vi "Run.vi"(8 "error in (no error)":errorcluster, 11 "Switching Times in":refnum<class "Switching Time.lvclass">) -> (0 "error out":errorcluster, 1 "Parameters":cluster{"Name":string, "Value":string}[](array[cluster]), 2 "Canceled":bool, 3 "Switching Times out":refnum<class "Switching Time.lvclass">)   [LabVIEW 2020, in "Switching Time.lvclass"]
doc: "This is the main test vi. It is here that the test is implemented."
uses:
  Switching Time.lvclass
  C:/Sandbox/Git_Sandbox/WiSpry Test Framework source code (LV20)/WiSpry Test Framework/Measurements/Measurement.lvclass
  Controls/Run States.ctl
  Devices/Controls/Change setting mode enum.ctl
  Measurement.lvclass/Measurement.ctl
  XML Handler/Controls/Result Cluster.ctl
  XML Handler/XML Handler.lvclass/XML Handler.ctl
  Support VI/Update parameters (array).vi
  Support VI/Update parameters (single).vi
  <vilib>/Waveform/WDTFileIO.llb/Export Waveforms To Spreadsheet File (1D).vi
  Measurement.lvclass
  Instruments/Signal Generator/Signal Generator.lvclass
  Devices/Device.lvclass
  Instruments/Oscilloscope/Oscilloscope.lvclass
  Instruments/Spectrum Analyzer/Spectrum Analyzer.lvclass
  Devices/PIC-device/PIC-Device.lvclass
  Instruments/Power Supply/Power Supply.lvclass
  Instruments/Digital Multimeter/Digital Multimeter.lvclass
  XML Handler/XML Handler.lvclass
panel:
  out "resulting string":string
  out "Waveform Graph":waveform(dbl)[](graph)
  in  "Cancel Button":bool
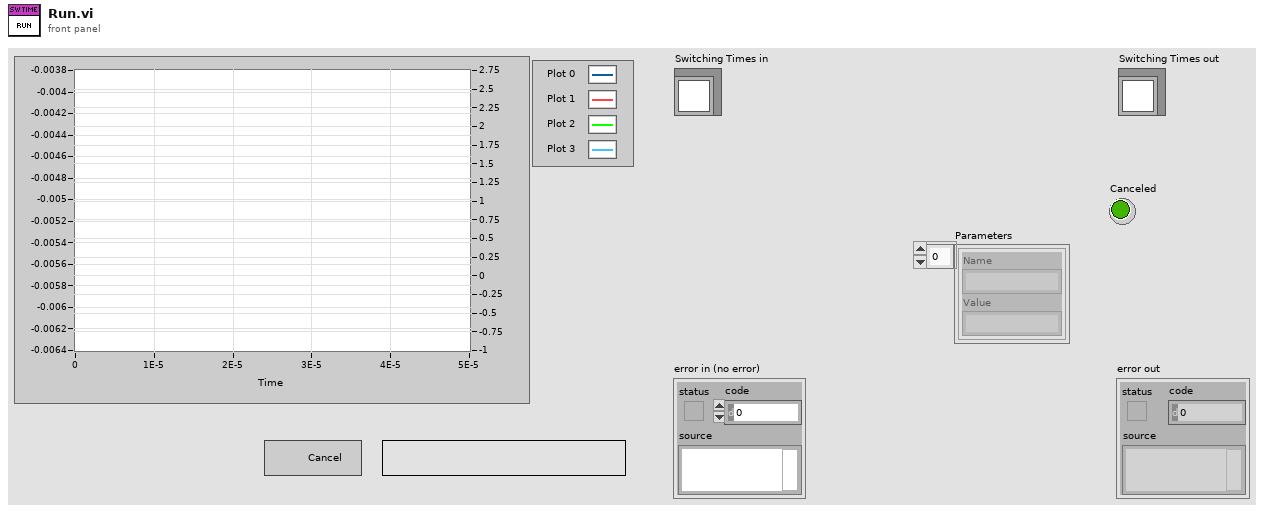
[diagram p1: front panel]
types:
  T1 = typedef "Measurement.lvclass/Run States.ctl" = enum16{"Init", "Set Device", "Read Environment", "Measure", "Done"}
  T2 = typedef "PIC-Device.lvclass/Change setting mode enum.ctl" = enum16{"Init", "Next", "Reset"}
  T3 = typedef "XML Handler.lvclass/Result Cluster.ctl" = cluster{"Name":string, "Value":string}
  T4 = typedef "Switching Time.lvclass/Method.ctl" = enum16{"Oscilloscope", "Spectrum Analyzer"}
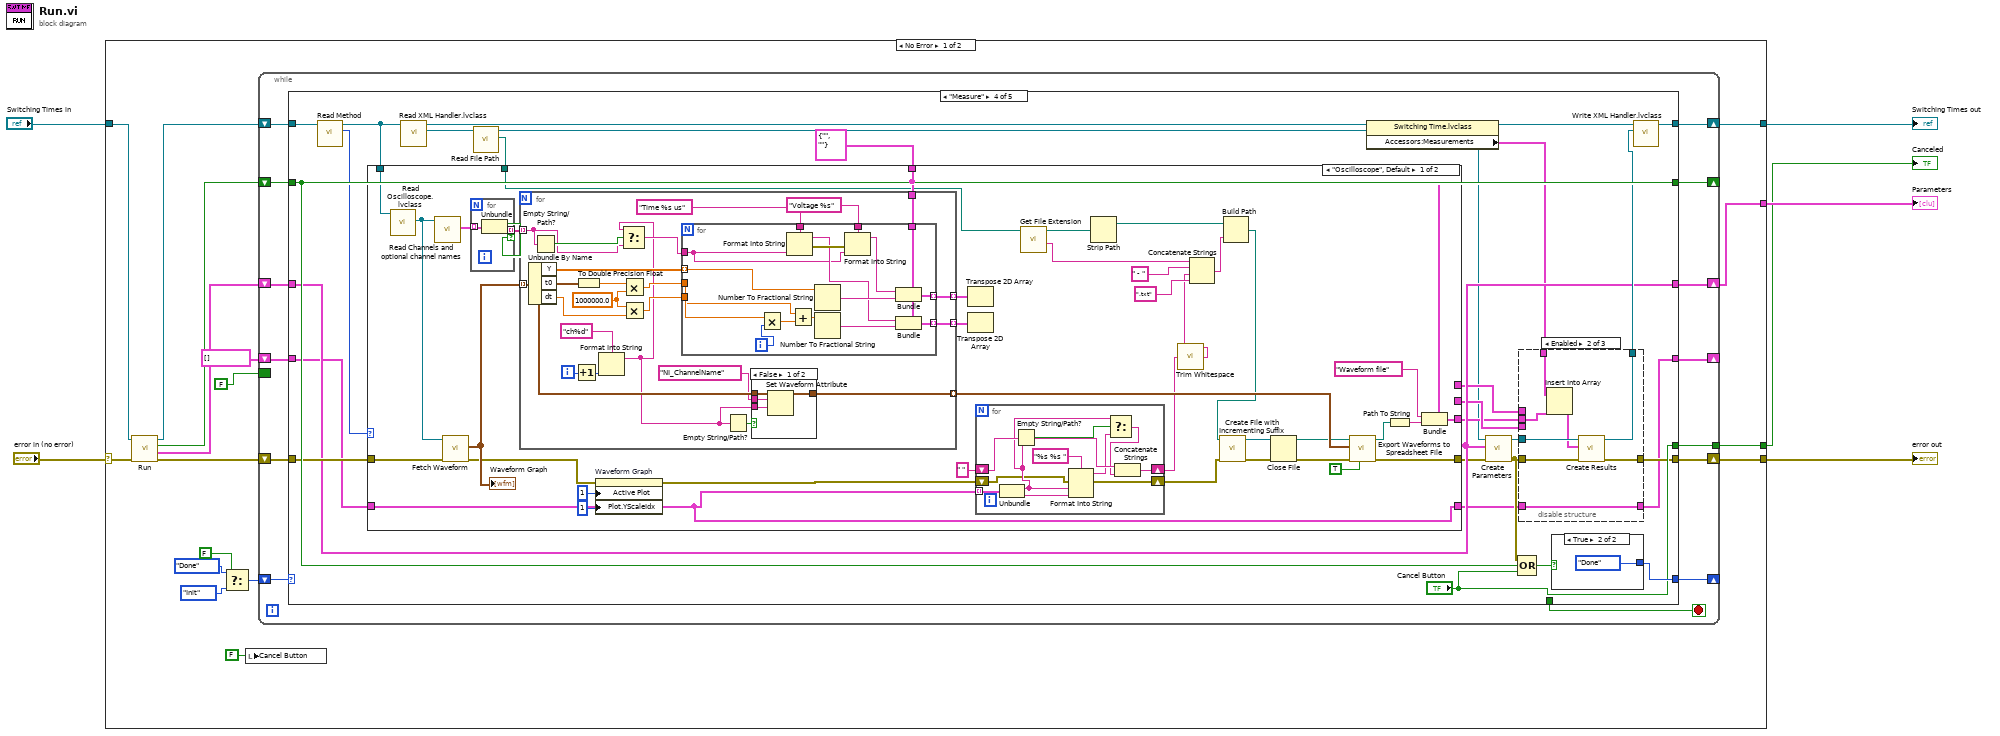
[diagram p0: block diagram]
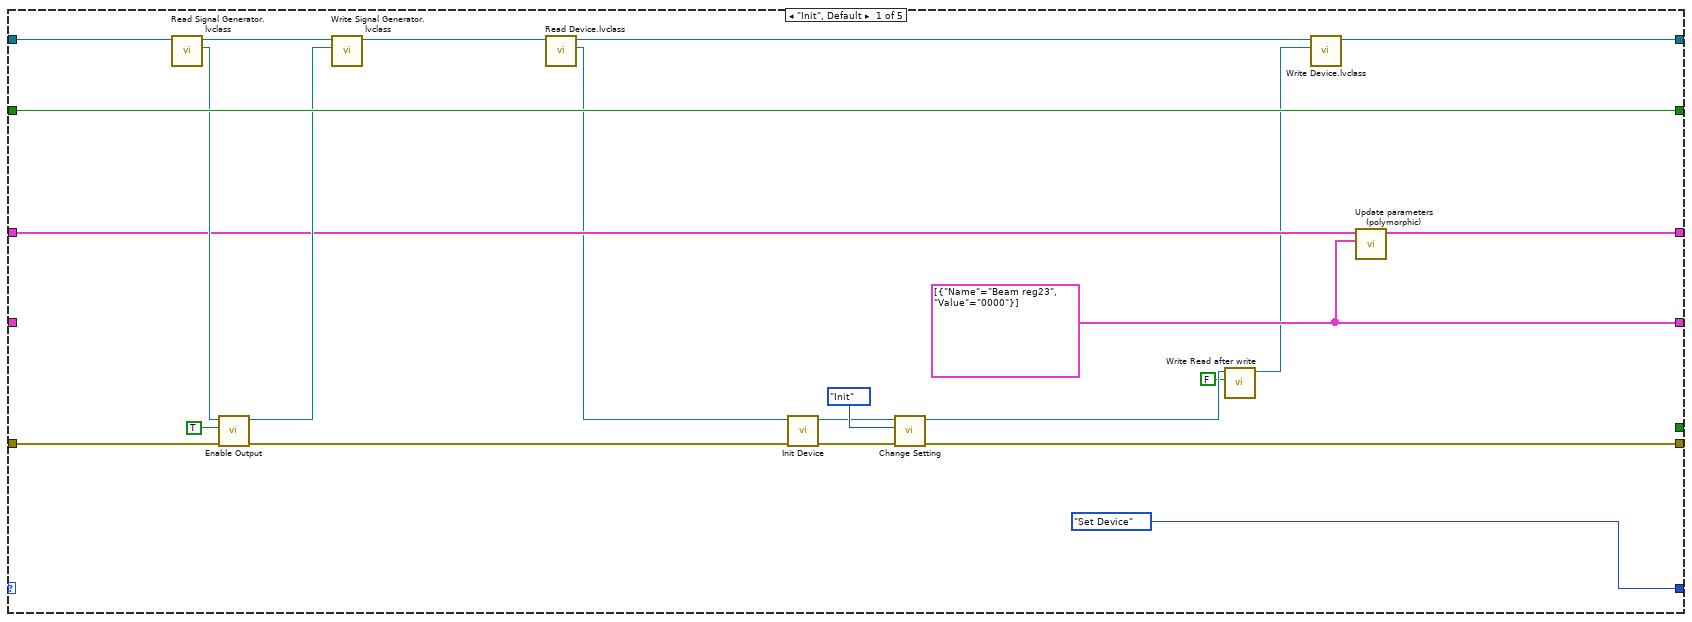
[diagram p2: hidden frame]
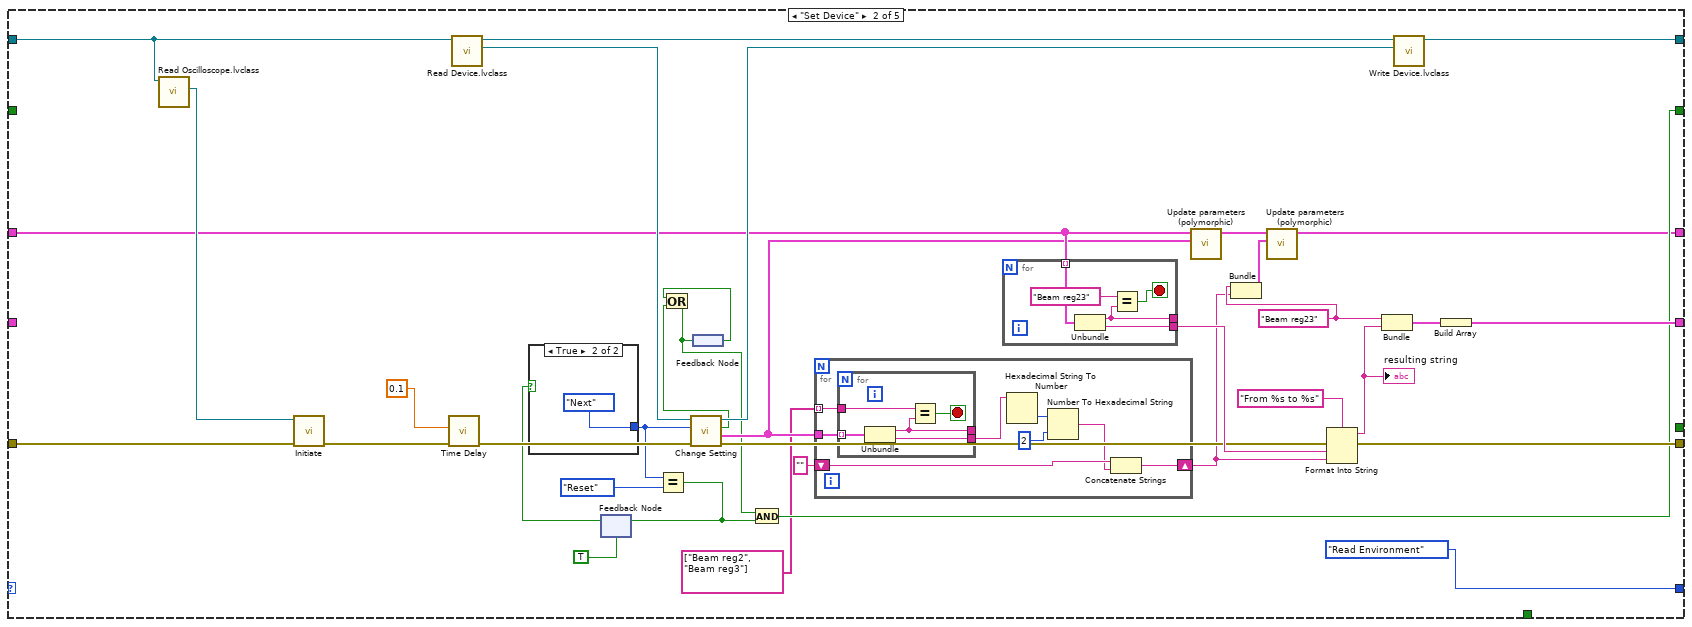
[diagram p3: hidden frame]
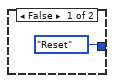
[diagram p4: hidden frame]
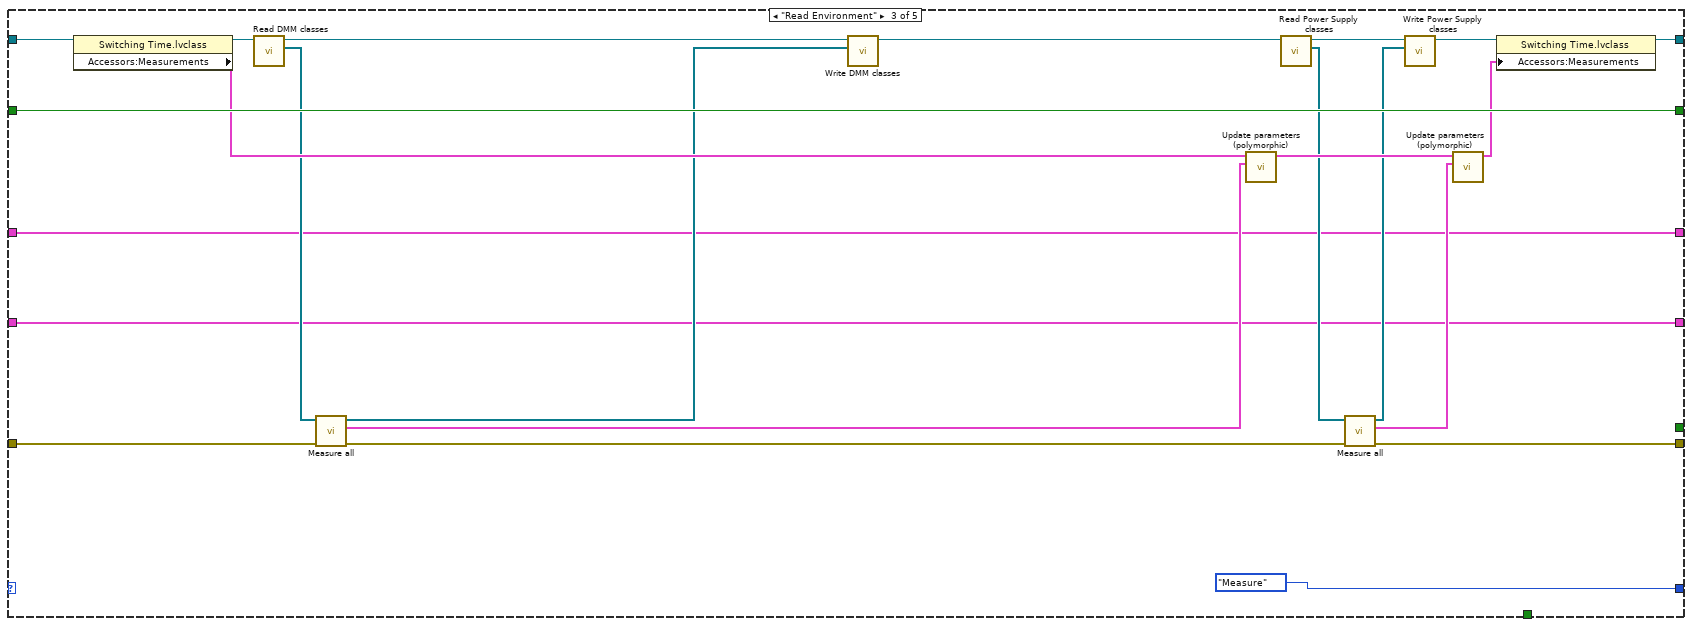
[diagram p5: hidden frame]
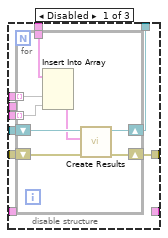
[diagram p6: hidden frame]
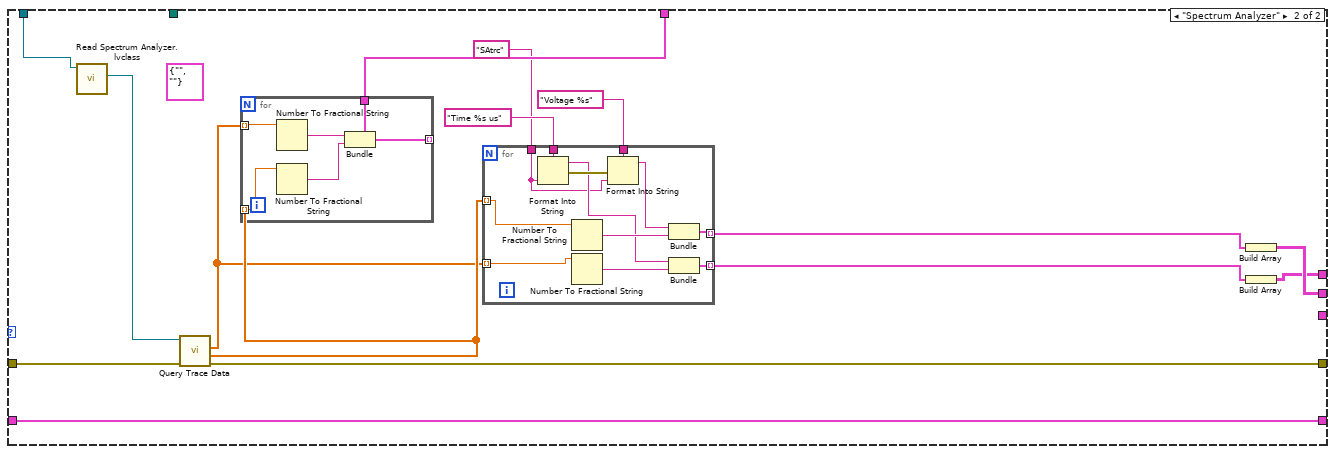
[diagram p9: hidden frame]
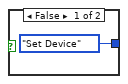
[diagram p10: hidden frame]
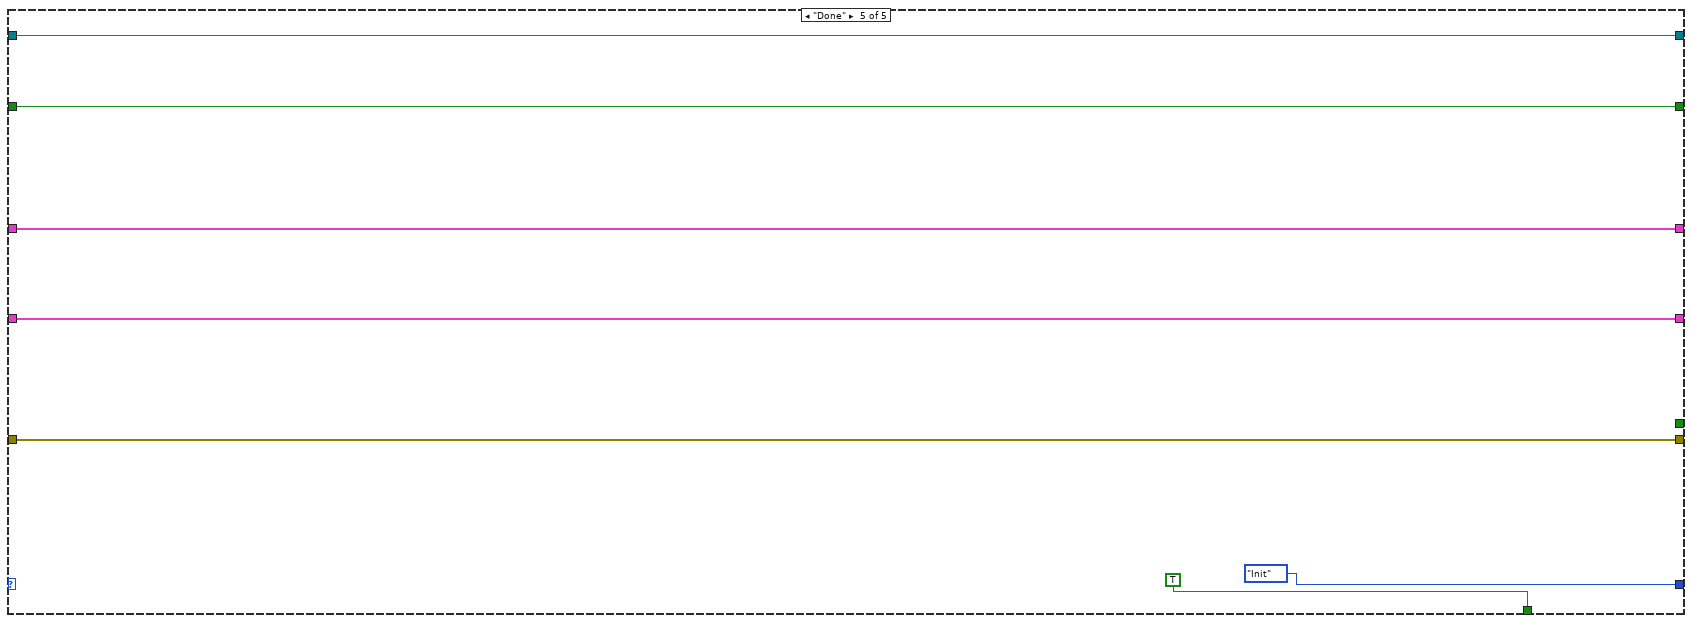
[diagram p11: hidden frame]
diagram:
  n1 = case shown="No Error" "error in (no error)" {
    selector: "error in (no error)" -> [w23 w329]
    tunnel: "Switching Times in" -> [w22 w328]
    tunnel: [w20 w329] -> w4
    tunnel: [w15 w328] -> w3
    tunnel: [w13 _] -> w1
    tunnel: [w11 _] -> w2
    frame No Error {
      n2 = call-parent "Run.vi"("error in (no error)"=w23, "Measurements in"=w22) -> ("error out"=w21:errorcluster, "Parameters"=w12:cluster{"Name":string, "Value":string}[], "Canceled"=w14:bool, "Measurements out"=w18:refnum<class "Switching Time.lvclass">)  [unwired: 6 in]
      n3 = Select(t=Run_States."Done" ("Run states"), s=FALSE, f=Run_States."Init" ("Run states")) -> (s? t:f=w16:T1)
      n4 = local write "Cancel Button"(FALSE ("Cancel Button")) -> ()
      n5 = while {
        shift-right: [w35] -> w20
        shift-left: w21 -> [w36]
        shift-right: [w34] -> w15
        shift-left: w18 -> [w33]
        shift-right: [w31] -> _
        shift-left: w16 -> [w37]
        tunnel: [w30] -> w13
        shift-right: [w26] -> w11
        shift-left: w12 -> [w28]
        shift-right: [w27] -> _
        shift-left: w14 -> [w29]
        shift-right: [w25] -> _
        shift-left: cluster{"Name":string, "Value":string}[] [] ("Changes") -> [w24]
        border: FALSE -> [_]
        stop <- w32 stop-if-true
        n6 = case shown="\"Measure\"" w37 {
          tunnel: w36 -> [w58 w91 w123 w162 w327]
          tunnel: [w49 w80 w124 w155 w327] -> w35
          tunnel: [w50 w92 w121 w158 w326] -> w34
          tunnel: w33 -> [w57 w90 w122 w161 w326]
          tunnel: [_ _ _ _ TRUE] -> w32
          tunnel: [Run_States."Set Device" ("Run states") Run_States."Read Environment" ("Run states") Run_States."Measure" ("Run states") w165 Run_States."Init" ("Run states")] -> w31
          tunnel: [_ _ _ "Cancel Button" _] -> w30
          tunnel: w29 -> [w59 _ w138 w163 w323]
          tunnel: w28 -> [w45 w78 w118 w156 w322]
          tunnel: [w59 w71 w138 w163 w323] -> w27
          tunnel: [w44 w67 w118 w156 w322] -> w26
          tunnel: [w43 w81 w117 w141 w321] -> w25
          tunnel: w24 -> [_ _ w117 w142 w321]
          frame "Init", Default {
            w43 = cluster{"Name":string, "Value":string}[] [{"Name"="Beam reg23", "Value"="0000"}] ("Changes")
            n7 = call-dynamic "Read Signal Generator.lvclass.vi"("Switching Time in"=w57) -> ("Signal Generator.lvclass"=w56:refnum<class "Signal Generator.lvclass">, "Switching Time out"=w55:refnum<class "Switching Time.lvclass">)  [unwired: 9 in]
            n8 = call-dynamic "Enable Output.vi"("error in (no error)"=w58, "Output Enable (F)"=TRUE, "Signal Generator in"=w56) -> ("error out"=w46:errorcluster, "Signal Generator out"=w54:refnum<class "Signal Generator.lvclass">)  [unwired: 7 in]
            n9 = call-dynamic "Write Signal Generator.lvclass.vi"("Signal Generator.lvclass"=w54, "Switching Time in"=w55) -> ("Switching Time out"=w51:refnum<class "Switching Time.lvclass">)  [unwired: 9 in]
            n10 = call "Read Device.lvclass.vi"("Measurements in"=w51) -> ("Device.lvclass"=w41:refnum<class "Device.lvclass">, "Measurements out"=w42:refnum<class "Switching Time.lvclass">)  [unwired: 9 in]
            n11 = call-dynamic "Init Device.vi"("error in (no error)"=w46, "Device in"=w41) -> ("error out"=w47:errorcluster, "Device out"=w48:refnum<class "Device.lvclass">)  [unwired: 8 in]
            n12 = call-dynamic "Change Setting.vi"("error in (no error)"=w47, "Change setting mode"=Change_setting_mode_enum."Init", "Device in"=w48) -> ("error out"=w49:errorcluster, "Device out"=w40:refnum<class "Device.lvclass">)  [unwired: 5 in, 2 out]
            n13 = call-dynamic "Write Read after write.vi"("Read after write"=FALSE, "Device in"=w40) -> ("Device out"=w39:refnum<class "Device.lvclass">)  [unwired: 9 in]
            n14 = call "Write Device.lvclass.vi"("Device.lvclass"=w39, "Measurements in"=w42) -> ("Measurements out"=w50:refnum<class "Switching Time.lvclass">)  [unwired: 9 in]
            n15 = call-poly "Update parameters (polymorphic).vi"("New Parameters"=w43, "Parameters"=w45) -> ("Parameters Out"=w44:cluster{"Name":string, "Value":string}[])  [unwired: 9 in]
          }
          frame "Set Device" {
            w66 = "Beam reg23" ("x")
            n16 = call-dynamic "Read Oscilloscope.lvclass.vi"("Switching Time in"=w90) -> ("Oscilloscope.lvclass"=w89:refnum<class "Oscilloscope.lvclass">)  [unwired: 9 in, 1 out]
            n17 = call-dynamic "Initiate.vi"("error in (no error)"=w91, "Oscilloscope in"=w89) -> ("error out"=w88:errorcluster)  [unwired: 8 in, 1 out]
            n18 = call "Time Delay"("error in (no error)"=w88, "Delay Time (s)"=0.1) -> ("error out"=w87:errorcluster)  [unwired: 9 in]
            n19 = call "Read Device.lvclass.vi"("Measurements in"=w90) -> ("Device.lvclass"=w95:refnum<class "Device.lvclass">, "Measurements out"=w93:refnum<class "Switching Time.lvclass">)  [unwired: 9 in]
            n20 = feedback #1(TRUE) -> (w74:bool)
            n21 = case shown="True" w74 {
              tunnel: [Change_setting_mode_enum."Reset" ("Change setting mode") Change_setting_mode_enum."Next" ("Change setting mode")] -> w75
              frame False {
              }
              frame True {
              }
            }
            n22 = Equal?(x=w75, y=Change_setting_mode_enum."Reset" ("Change setting mode")) -> (x = y?=w72:bool)
            n23 = feedback-in #1(w72) -> ()
            n24 = call-dynamic "Change Setting.vi"("error in (no error)"=w87, "Change setting mode"=w75, "Device in"=w95) -> ("error out"=w79:errorcluster, "Changes"=w77:cluster{"Name":string, "Value":string}[], "Last setting"=w63:bool, "Device out"=w94:refnum<class "Device.lvclass">)  [unwired: 5 in]
            n25 = feedback #2() -> (w62:bool)
            n26 = Or(x=w62, y=w63) -> (x .or. y?=w61:bool)
            n27 = feedback-in #2(w61) -> ()
            n28 = And(x=w61, y=w72) -> (x .and. y?=w71:bool)
            n29 = for {
              tunnel: w77 -> [w104]
              tunnel: string[] ["Beam reg2", "Beam reg3"] -> [w103] mode=indexing
              shift-right: [w102] -> w65
              shift-left: "" -> [w101]
              n30 = for {
                tunnel: [w107] -> _
                tunnel: [w109] -> w98
                tunnel: w104 -> [w108] mode=indexing
                tunnel: w103 -> [w105]
                stop <- w106 stop-if-true
                n31 = Unbundle(w108) -> ("Name"=w107:string, "Value"=w109:string)
                n32 = Equal?(x=w105, y=w107) -> (x = y?=w106:bool)
              }
              n33 = Hexadecimal String To Number(string=w98) -> (number=w100:u32)  [unwired: 2 in, 1 out]
              n34 = Number To Hexadecimal String(1:i16 2 ("width (-)"), 2:w100) -> (0:w97:string)
              n35 = Concatenate Strings(w101, w97) -> (w102:string)
            }
            n36 = for {
              tunnel: [w114] -> _
              tunnel: [w116] -> w84
              tunnel: w78 -> [w115] mode=indexing
              stop <- w112 stop-if-true
              n37 = Unbundle(w115) -> ("Name"=w114:string, "Value"=w116:string)
              n38 = Equal?(x="Beam reg23", y=w114) -> (x = y?=w112:bool)
            }
            n39 = call-poly "Update parameters (polymorphic).vi"("New Parameters"=w77, "Parameters"=w78) -> ("Parameters Out"=w68:cluster{"Name":string, "Value":string}[])  [unwired: 9 in]
            n40 = Bundle("x"=w66, w65) -> (w64:cluster{"x":string, string})  [unwired: 1 in]
            n41 = call-poly "Update parameters (polymorphic).vi"("New Parameter"=w64, "Parameters"=w68) -> ("Parameters Out"=w67:cluster{"Name":string, "Value":string}[])  [unwired: 9 in]
            n42 = Format Into String(format string="From %s to %s", error in=w79, w84, w65) -> (resulting string=w83:string, error out=w80:errorcluster)  [unwired: 1 in]
            "resulting string" <- w83
            n43 = Bundle("x"=w66, w83) -> (w82:cluster{"x":string, string})  [unwired: 1 in]
            n44 = call "Write Device.lvclass.vi"("Device.lvclass"=w94, "Measurements in"=w93) -> ("Measurements out"=w92:refnum<class "Switching Time.lvclass">)  [unwired: 9 in]
            n45 = Build Array(w82) -> (w81:cluster{"x":string, string}[])
          }
          frame "Read Environment" {
            n46 = property class="Switching Time.lvclass"(reference=w122) -> (reference out=w134:refnum<class "Switching Time.lvclass">, "Accessors:Measurements"=w135:cluster{"Name":string, "Value":string}[])  [unwired: 1 in, 1 out]
            n47 = call-dynamic "Read DMM classes.vi"("Measurements in"=w134) -> ("DMM classes"=w130:refnum<class "Digital Multimeter.lvclass">[], "Measurements out"=w125:refnum<class "Switching Time.lvclass">)  [unwired: 9 in]
            n48 = call "Measure all.vi"("error in (no error)"=w123, "Digital Multimeters in"=w130) -> ("error out"=w132:errorcluster, "Measurements"=w119:T3[], "Digital Multimeters out"=w131:refnum<class "Digital Multimeter.lvclass">[])  [unwired: 5 in, 2 out]
            n49 = call-dynamic "Write DMM classes.vi"("DMM classes"=w131, "Measurements in"=w125) -> ("Measurements out"=w129:refnum<class "Switching Time.lvclass">)  [unwired: 9 in]
            n50 = call-poly "Update parameters (polymorphic).vi"("New Parameters"=w119, "Parameters"=w135) -> ("Parameters Out"=w133:cluster{"Name":string, "Value":string}[])  [unwired: 9 in]
            n51 = call-dynamic "Read Power Supply classes.vi"("Measurements in"=w129) -> ("Power Supply classes"=w127:refnum<class "Power Supply.lvclass">[], "Measurements out"=w126:refnum<class "Switching Time.lvclass">)  [unwired: 9 in]
            n52 = call "Measure all.vi"("error in (no error)"=w132, "Power Supplies in"=w127) -> ("error out"=w124:errorcluster, "Measurements"=w120:T3[], "Power Supplies out"=w128:refnum<class "Power Supply.lvclass">[])  [unwired: 5 in, 2 out]
            n53 = call-dynamic "Write Power Supply classes.vi"("Power Supply classes"=w128, "Measurements in"=w126) -> ("Measurements out"=w136:refnum<class "Switching Time.lvclass">)  [unwired: 9 in]
            n54 = call-poly "Update parameters (polymorphic).vi"("New Parameters"=w120, "Parameters"=w133) -> ("Parameters Out"=w137:cluster{"Name":string, "Value":string}[])  [unwired: 9 in]
            n55 = property class="Switching Time.lvclass"(reference=w136, "Accessors:Measurements"=w137) -> (reference out=w121:refnum<class "Switching Time.lvclass">)  [unwired: 1 in, 1 out]
          }
          frame "Measure" {
            n56 = call-dynamic "Read Method.vi"("Switching Time in"=w161) -> ("Method"=w160:T4, "Switching Time out"=w154:refnum<class "Switching Time.lvclass">)  [unwired: 9 in]
            n57 = call "Read XML Handler.lvclass.vi"("Measurements in"=w154) -> ("XML Handler.lvclass"=w144:refnum<class "XML Handler.lvclass">, "Measurements out"=w147:refnum<class "Switching Time.lvclass">)  [unwired: 9 in]
            n58 = call "Read File Path.vi"("XML Handler in"=w144) -> ("File Path"=w143:path, "XML Handler out"=w145:refnum<class "XML Handler.lvclass">)  [unwired: 9 in]
            n59 = case shown="\"Oscilloscope\", Default" w160 {
              tunnel: w162 -> [w226 w300]
              tunnel: [w218 w299] -> w148
              tunnel: w154 -> [w225 w298]
              tunnel: T3 {"Name"="", "Value"=""} ("Result Cluster") -> [w217 w296]
              tunnel: [_ w289] -> w152
              tunnel: [_ w287] -> w151
              tunnel: [w213 _] -> w146
              tunnel: w143 -> [w198 _]
              tunnel: w142 -> [w205 w286]
              tunnel: [w205 w286] -> w140
              frame "Oscilloscope", Default {
                n60 = call-dynamic "Read Oscilloscope.lvclass.vi"("Switching Time in"=w225) -> ("Oscilloscope.lvclass"=w224:refnum<class "Oscilloscope.lvclass">)  [unwired: 9 in, 1 out]
                n61 = call-dynamic "Read Channels and optional channel names.vi"("Oscilloscope in"=w224) -> ("Channels and optional channel names"=w223:cluster{"Enabled":bool, "Channel name":string}[])  [unwired: 9 in, 1 out]
                n62 = call-dynamic "Fetch Waveform.vi"("error in (no error)"=w226, "Oscilloscope in"=w224) -> ("error out"=w192:errorcluster, "Waveform Data"=w221:waveform(dbl)[])  [unwired: 7 in, 1 out]
                "Waveform Graph" <- w221
                n63 = for {
                  tunnel: w223 -> [w240] mode=indexing
                  tunnel: [w239] -> w222 mode=indexing if=w238
                  n64 = Unbundle(w240) -> ("Enabled"=w238:bool, "Channel name"=w239:string)
                }
                n65 = for {
                  tunnel: w221 -> [w244] mode=indexing
                  tunnel: [w261] -> w219 mode=indexing
                  tunnel: [w260] -> w220 mode=indexing
                  tunnel: w217 -> [w259]
                  tunnel: w222 -> [w252] mode=indexing
                  tunnel: [w242] -> w212 mode=indexing
                  i -> [w255]
                  w246 = 1000000.0 ("y")
                  n66 = Unbundle By Name(w244) -> ("Y"=w263:dbl[], "t0"=w262:timestamp, "dt"=w249:dbl)
                  n67 = Empty String/Path?(string/path=w252) -> (empty?=w253:bool)
                  n68 = Increment(x=w255) -> (x+1=w254:i32)
                  n69 = To Double Precision Float(number=w262) -> (double precision float=w250:dbl)
                  n70 = Format Into String(format string="ch%d", w254) -> (resulting string=w243:string)  [unwired: 2 in, 1 out]
                  n71 = Select(t=w243, s=w253, f=w252) -> (s? t:f=w251:string)
                  n72 = Multiply(x=w250, y=w246) -> (x*y=w247:dbl)
                  n73 = Multiply(x=w246, y=w249) -> (x*y=w248:dbl)
                  n74 = for {
                    tunnel: w263 -> [w285] mode=indexing
                    tunnel: w259 -> [w269]
                    tunnel: w248 -> [w283]
                    tunnel: w247 -> [w280]
                    tunnel: [w279] -> w261 mode=indexing
                    tunnel: [w278] -> w260 mode=indexing
                    tunnel: "Time %s us" ("format string") -> [w275]
                    tunnel: w251 -> [w270]
                    tunnel: "Voltage %s" ("format string") -> [w272]
                    i -> [w282]
                    n75 = Multiply(x=w283, y=w282) -> (x*y=w284:dbl)
                    n76 = Format Into String(format string=w275, w270) -> (resulting string=w273:string, error out=w274:errorcluster)  [unwired: 2 in]
                    n77 = Add(x=w280, y=w284) -> (x+y=w281:dbl)
                    n78 = Number To Fractional String(number=w285) -> (F-format string=w277:string)  [unwired: 3 in]
                    n79 = Number To Fractional String(number=w281) -> (F-format string=w276:string)  [unwired: 3 in]
                    n80 = Format Into String(format string=w272, error in=w274, w270) -> (resulting string=w271:string)  [unwired: 1 in, 1 out]
                    n81 = Bundle(cluster=w269, "Name"=w271, "Value"=w277) -> (w278:T3)
                    n82 = Bundle(cluster=w269, "Name"=w273, "Value"=w276) -> (w279:T3)
                  }
                  n83 = Empty String/Path?(string/path=w243) -> (empty?=w245:bool)
                  n84 = case shown="False" w245 {
                    tunnel: w244 -> [w267 w268]
                    tunnel: "NI_ChannelName" ("name") -> [w266 _]
                    tunnel: [w265 w268] -> w242
                    tunnel: w243 -> [w264 _]
                    frame False {
                      n85 = Set Waveform Attribute(5:w264, 6:w266, 7:w267) -> (3:w265:waveform(dbl))  [unwired: 1 in, 2 out]
                    }
                    frame True {
                    }
                  }
                }
                n86 = property on="Waveform Graph" class="WFGraph (strict)"(error in=w192, "Active Plot"=u32 1, "Plot.YScaleIdx"=u32 1 ("Plot.Y Scale Index")) -> (error out=w191:errorcluster)  [unwired: 1 in, 1 out]
                n87 = Transpose 2D Array(2D array=w220) -> ()  [unwired: 1 out]
                n88 = Transpose 2D Array(2D array=w219) -> ()  [unwired: 1 out]
                n89 = for {
                  tunnel: w205 -> [w237] mode=indexing
                  shift-right: [w234] -> w196
                  shift-left: " " -> [w235]
                  shift-right: [w233] -> w203
                  shift-left: w191 -> [w227]
                  n90 = Unbundle(w237) -> ("Name"=w231:string, "Value"=w228:string)
                  n91 = Empty String/Path?(string/path=w231) -> (empty?=w232:bool)
                  n92 = Format Into String(format string="%s %s ", error in=w227, w231, w228) -> (resulting string=w230:string, error out=w233:errorcluster)  [unwired: 1 in]
                  n93 = Select(t=w231, s=w232, f=w230) -> (s? t:f=w229:string)
                  n94 = Concatenate Strings(w235, w229) -> (w234:string)
                }
                n95 = call <vilib>:"Get File Extension.vi"("file"=w198) -> ("filename without extension"=w201:string, "dup file"=w197:path)  [unwired: 6 in, 3 out]
                n96 = Strip Path(path=w197) -> (stripped path=w202:path)  [unwired: 1 out]
                n97 = call <vilib>:"Trim Whitespace.vi"("string"=w196) -> ("trimmed string"=w195:string)  [unwired: 1 in]
                n98 = Concatenate Strings(w201, " - " ("string"), w195, ".txt" ("string")) -> (w200:string)
                n99 = Build Path(base path=w202, name or relative path=w200) -> (appended path=w206:path)
                n100 = call <vilib>:"Create File with Incrementing Suffix.vi"("error in (no error)"=w203, "file path"=w206) -> ("error out"=w208:errorcluster, "refnum out"=w211:refnum<file>)  [unwired: 7 in, 1 out]
                n101 = Close File(refnum=w211, error in=w208) -> (path=w210:path, error out=w209:errorcluster)
                n102 = call-poly <vilib>:"Export Waveforms to Spreadsheet File.vi"("append to file? (new file:F)"=TRUE, "error in (no error)"=w209, "waveforms"=w212, "file path (dialog if empty)"=w210) -> ("error out"=w218:errorcluster, "new file path (Not A Path if cancelled)"=w215:path)  [unwired: 6 in]
                n103 = Path To String(path=w215) -> (string=w214:string)
                n104 = Bundle(cluster=w217, "Name"="Waveform file", "Value"=w214) -> (w213:T3)
              }
              frame "Spectrum Analyzer" {
                (unwired) T3 {"Name"="", "Value"=""} ("Result Cluster")
                n105 = call-dynamic "Read Spectrum Analyzer.lvclass.vi"("Switching Time in"=w298) -> ("Spectrum Analyzer.lvclass"=w297:refnum<class "Spectrum Analyzer.lvclass">)  [unwired: 9 in, 1 out]
                n106 = call-dynamic "Query Trace Data.vi"("error in (no error)"=w300, "Spectrum Analyzer in"=w297) -> ("error out"=w299:errorcluster, "Level"=w293:dbl[], "Frequency/Time"=w292:dbl[])  [unwired: 6 in, 1 out]
                n107 = for {
                  tunnel: w292 -> [w316] mode=indexing
                  tunnel: w293 -> [w317] mode=indexing
                  tunnel: w296 -> [w318]
                  tunnel: [w313] -> _ mode=indexing
                  n108 = Number To Fractional String(number=w316) -> (F-format string=w315:string)  [unwired: 3 in]
                  n109 = Number To Fractional String(number=w317) -> (F-format string=w314:string)  [unwired: 3 in]
                  n110 = Bundle(cluster=w318, "Name"=w315, "Value"=w314) -> (w313:T3)
                }
                n111 = for {
                  tunnel: w293 -> [w312] mode=indexing
                  tunnel: [w311] -> w288 mode=indexing
                  tunnel: [w310] -> w290 mode=indexing
                  tunnel: "Time %s us" ("format string") -> [w307]
                  tunnel: "Voltage %s" ("format string") -> [w304]
                  tunnel: w292 -> [w302] mode=indexing
                  tunnel: "SAtrc" ("format string") -> [w301]
                  n112 = Format Into String(format string=w307, w301) -> (resulting string=w305:string, error out=w306:errorcluster)  [unwired: 2 in]
                  n113 = Number To Fractional String(number=w312) -> (F-format string=w309:string)  [unwired: 3 in]
                  n114 = Number To Fractional String(number=w302) -> (F-format string=w308:string)  [unwired: 3 in]
                  n115 = Format Into String(format string=w304, error in=w306, w301) -> (resulting string=w303:string)  [unwired: 1 in, 1 out]
                  n116 = Bundle(w303, w309) -> (w310:cluster{string, string})  [unwired: 1 in]
                  n117 = Bundle(w305, w308) -> (w311:cluster{string, string})  [unwired: 1 in]
                }
                n118 = Build Array(w290) -> (w289:cluster{string, string}[][])
                n119 = Build Array(w288) -> (w287:cluster{string, string}[][])
              }
            }
            n120 = property class="Switching Time.lvclass"(reference=w147) -> (reference out=w159:refnum<class "Switching Time.lvclass">, "Accessors:Measurements"=w150:cluster{"Name":string, "Value":string}[])  [unwired: 1 in, 1 out]
            n121 = call "Create Parameters.vi"("error in (no error)"=w148, "Parameters"=w156, "XML Handler in"=w145) -> ("XML Handler out"=w149:refnum<class "XML Handler.lvclass">)  [unwired: 7 in, 1 out]
            n122 = Compound Arithmetic op=OR(w148, w163, "Cancel Button") -> (w166:bool)
            n123 = disable-structure shown="Enabled" {
              disable-tunnel: [w173 w189 _] -> w157
              disable-tunnel: [w172 w188 _] -> w155
              disable-tunnel: w152 -> [w171 _ _]
              disable-tunnel: w151 -> [w170 _ _]
              disable-tunnel: w150 -> [w169 w187 _]
              disable-tunnel: w149 -> [w168 w186 _]
              disable-tunnel: w148 -> [w167 w185 _]
              disable-tunnel: w146 -> [_ w183 _]
              disable-tunnel: [_ w182 _] -> w141
              disable-tunnel: w140 -> [_ w182 _]
              frame Disabled {
                n124 = for {
                  tunnel: w171 -> [w174] mode=indexing
                  tunnel: w170 -> [w175] mode=indexing
                  tunnel: w169 -> [w179]
                  shift-right: [w181] -> w173
                  shift-left: w168 -> [w178]
                  shift-right: [w180] -> w172
                  shift-left: w167 -> [w177]
                  n125 = Insert Into Array(array=w179, new element #1=w175, new element #2=w174) -> (w176:cluster{"Name":string, "Value":string}[])  [unwired: 1 in]
                  n126 = call "Create Results.vi"("error in (no error)"=w177, "Results"=w176, "XML Handler in"=w178) -> ("error out"=w180:errorcluster, "XML Handler out"=w181:refnum<class "XML Handler.lvclass">)  [unwired: 7 in]
                }
              }
              frame Enabled {
                n127 = Insert Into Array(array=w187, new element=w183) -> (w184:cluster{"Name":string, "Value":string}[])  [unwired: 1 in]
                n128 = call "Create Results.vi"("error in (no error)"=w185, "Results"=w184, "XML Handler in"=w186) -> ("error out"=w188:errorcluster, "XML Handler out"=w189:refnum<class "XML Handler.lvclass">)  [unwired: 7 in]
              }
              frame Disabled {
              }
            }
            n129 = case shown="True" w166 {
              tunnel: [Run_States."Set Device" Run_States."Done"] -> w165
              frame False {
              }
              frame True {
              }
            }
            n130 = call "Write XML Handler.lvclass.vi"("XML Handler.lvclass"=w157, "Measurements in"=w159) -> ("Measurements out"=w158:refnum<class "Switching Time.lvclass">)  [unwired: 9 in]
          }
          frame "Done" {
          }
        }
      }
    }
    frame Error {
    }
  }
  "error out" <- w4
  "Switching Times out" <- w3
  "Canceled" <- w1
  "Parameters" <- w2
